vi "Weighted_Cross_Moments_TF.vi"(0 "Cluster 1":T1={"Colour"=0, "Inst type"=enum."Pitot-static tube", "Inst name"="Manometer voltage", "Symbol"="U", "Code name"="", "Extra Info"="U", "Inst Array"=enum."PWA", "Index"=0, "Voltage Index"=0, "Extra Titles"=[], "Extra Values"=[], "Eng Values"=[], "Time (ms)"=[], "TT / Voltage"=[], "U"=0.0, "u^2"=0.0, "u^3"=0.0, "u^4"=0.0, "Skew_u"=0.0, "Kurt_u"=0.0, "Mean % Err"=0.0, "% u'/U"=0.0} {"Skew_u" format="%.2f"; "% u'/U" format="%.2f"; "Mean % Err" format="%.2f"; "Kurt_u" format="%.2f"; "u^4" format="%.2f"; "u^3" format="%.2f"; "U" format="%.2f"; "u^2" format="%.2f"}, 1 "Cluster 2":T1={"Colour"=0, "Inst type"=enum."Pitot-static tube", "Inst name"="Manometer voltage", "Symbol"="U", "Code name"="", "Extra Info"="U", "Inst Array"=enum."PWA", "Index"=0, "Voltage Index"=0, "Extra Titles"=[], "Extra Values"=[], "Eng Values"=[], "Time (ms)"=[], "TT / Voltage"=[], "U"=0.0, "u^2"=0.0, "u^3"=0.0, "u^4"=0.0, "Skew_u"=0.0, "Kurt_u"=0.0, "Mean % Err"=0.0, "% u'/U"=0.0} {"Skew_u" format="%.2f"; "% u'/U" format="%.2f"; "Mean % Err" format="%.2f"; "Kurt_u" format="%.2f"; "u^4" format="%.2f"; "u^3" format="%.2f"; "U" format="%.2f"; "u^2" format="%.2f"}, 5 "Shift in":dbl[](array[numeric]) format="%.2f") -> (14 "Headers":string[](array[string]), 15 "Results":string[](array[string]), 19 "Shift out":dbl[](array[numeric]) format="%.2f")   [LabVIEW 2011]
uses:
  Controls/Analysis_info_cluster.ctl
  Controls/Inst_type.ctl
  Controls/Instrument_Array.ctl
  Globals/Meas_global.vi
panel:
  out "appended array":string[][](array[string])
  in  "Publish all results?":bool=TRUE
  in  "interp. method":i32(ring) items=["nearest", "linear", "spline", "cubic Hermite", "Lagrange"]
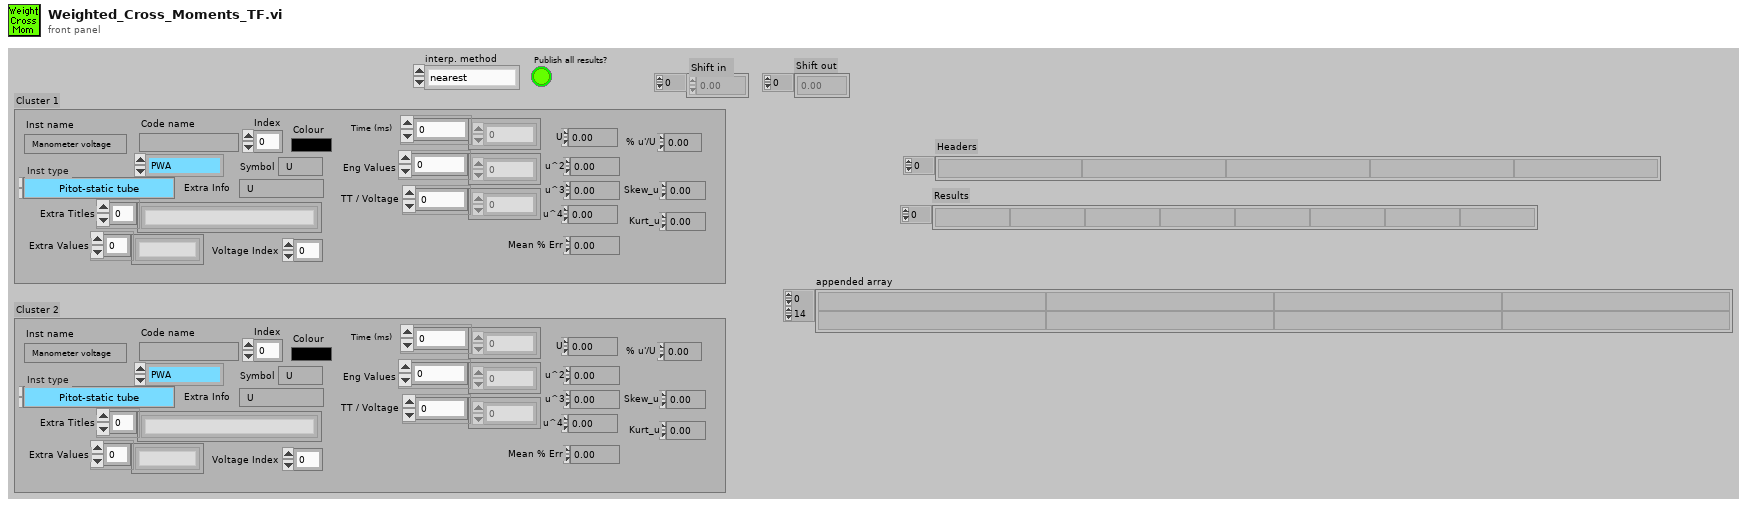
[diagram p1: front panel]
types:
  T1 = typedef "Analysis_info_cluster.ctl" = cluster{"Colour":u32, "Inst type":T2, "Inst name":string, "Symbol":string, "Code name":string, "Extra Info":string, "Inst Array":T3, "Index":i32, "Voltage Index":i32, "Extra Titles":string[], "Extra Values":string[], "Eng Values":dbl[], "Time (ms)":dbl[], "TT / Voltage":dbl[], "U":dbl, "u^2":dbl, "u^3":dbl, "u^4":dbl, "Skew_u":dbl, "Kurt_u":dbl, "Mean % Err":dbl, "% u'/U":dbl}
  T2 = typedef "Inst_type.ctl" = enum16{"Propeller anemometer", "Raw voltage", "Pressure Transducer", "Pitot-static tube", "Preston tube", "Hot wire", "Cross wire 1", "Cross wire 2", "Generic Linear", "Generic Polynomial", "Generic BackPoly", "Fast FID", "Thermocouple", "Cold wire", "Pulsed Wire", "LDA Vel", "LDA Tran time", "LDA Arr time"}
  T3 = typedef "Instrument_Array.ctl" = enum16{"PWA", "LDA", "Analogue"}
  T4 = enum16{"Mean only", "2nd Order Stats", "4th Order Stats"}
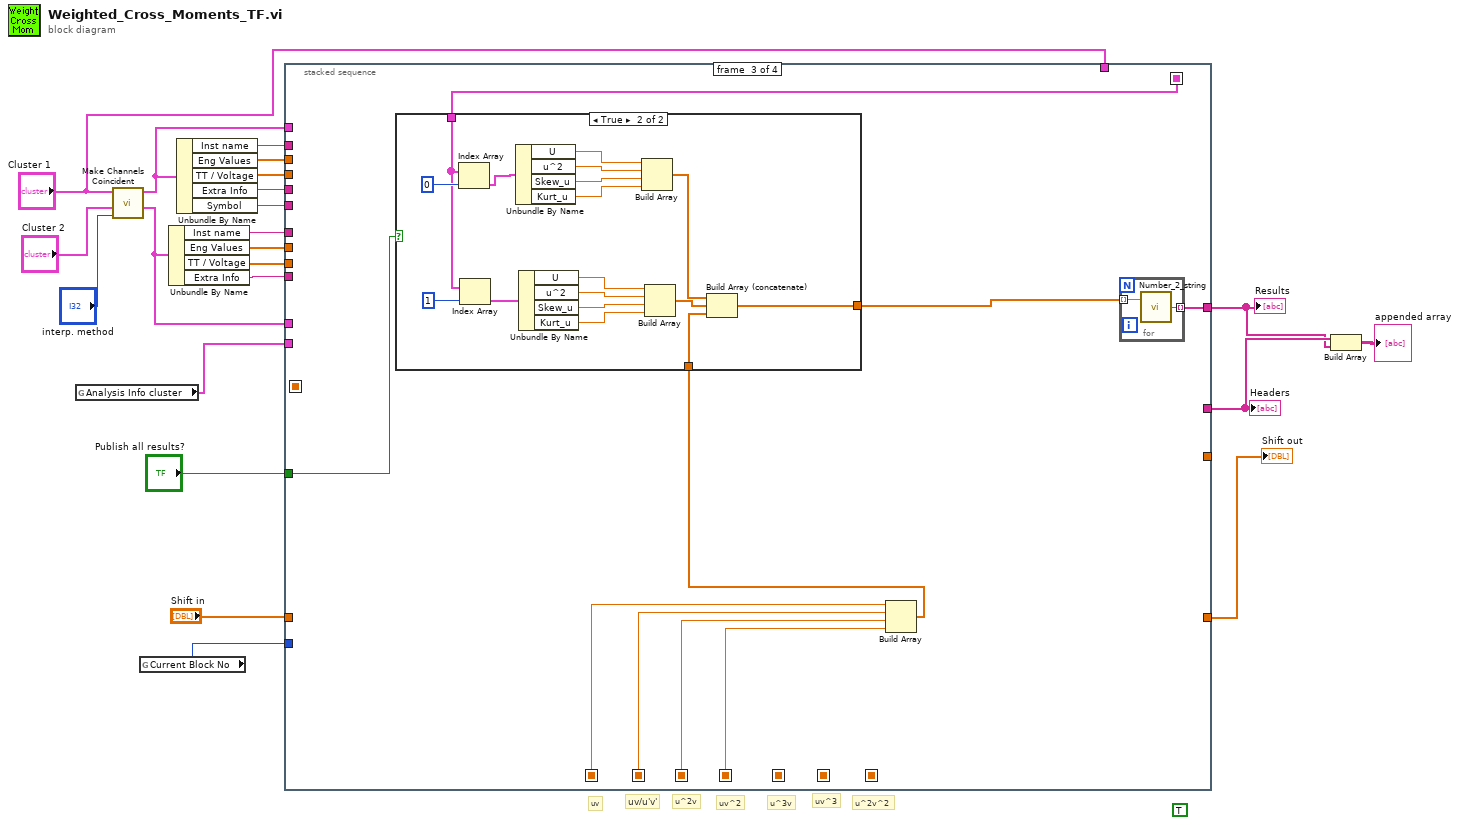
[diagram p0: block diagram]
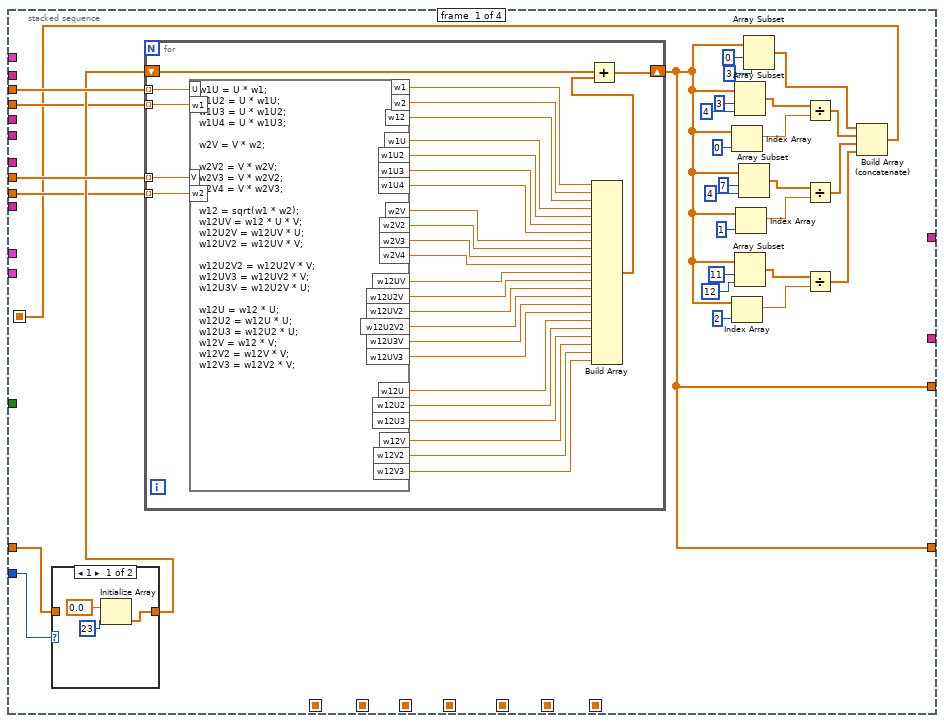
[diagram p2: hidden frame]
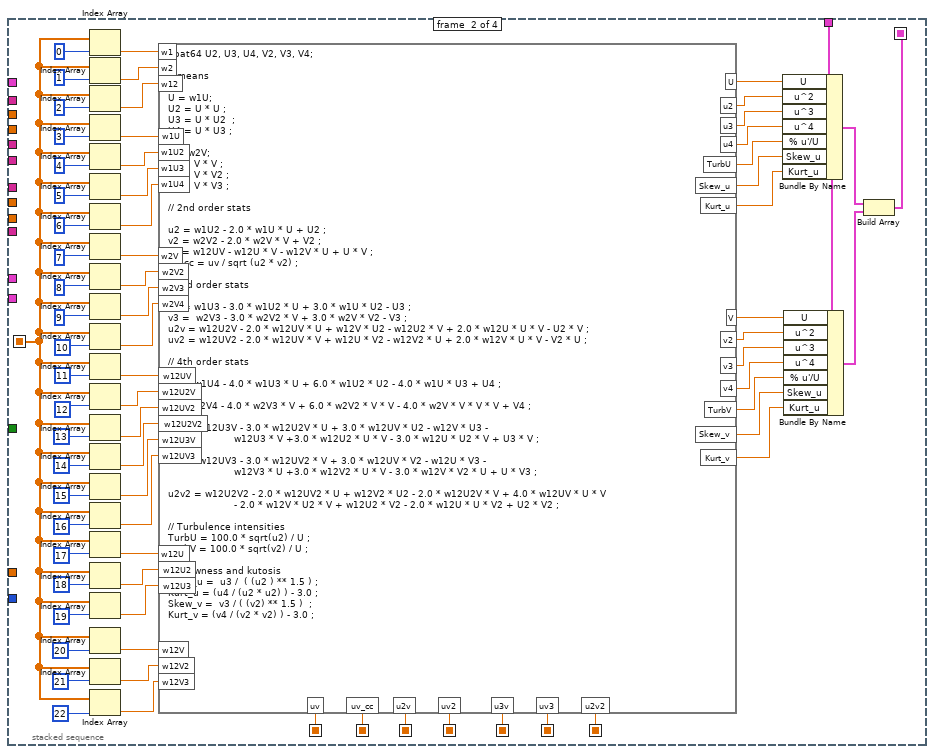
[diagram p4: hidden frame]
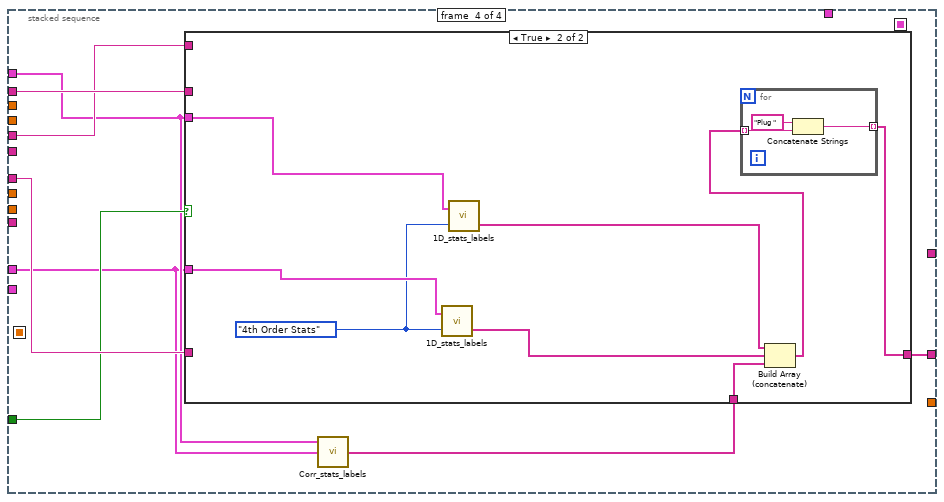
[diagram p6: hidden frame]
diagram:
  (unwired) TRUE
  # "u^2v^2"
  # "uv^3"
  # "u^3v"
  # "uv^2"
  # "u^2v"
  # "uv/u'v'"
  # "uv"
  n1 = global read "Meas_global.vi" "Analysis Info cluster"() -> (w18:T1[])
  n2 = call "Make Channels Coincident.vi"("interp. method"="interp. method", "Cluster 2"="Cluster 2", "Cluster 1"="Cluster 1") -> ("Coincident Channel 2"=w1:T1, "Coincident Channel 1"=w2:T1)  [unwired: 7 in]
  n3 = global read "Meas_global.vi" "Current Block No"() -> (w6:i32)
  n4 = Unbundle By Name(w1) -> ("Inst name"=w14:string, "Eng Values"=w20:dbl[], "TT / Voltage"=w21:dbl[], "Extra Info"=w17:string)
  n5 = Unbundle By Name(w2) -> ("Inst name"=w15:string, "Eng Values"=w19:dbl[], "TT / Voltage"=w22:dbl[], "Extra Info"=w16:string, "Symbol"=w3:string)
  n6 = stacked-sequence {
    seq-local: [_ w146 _ _] -> [_ _ w167 _]
    seq-local: [_ w145 _ _] -> [_ _ w166 _]
    seq-local: [w45 _ _ _] -> [_ w91 _ _]
    seq-local: [_ w140 _ _] -> [_ _ w165 _]
    seq-local: [_ w139 _ _] -> [_ _ w164 _]
    seq-local: [_ w87 _ _] -> [_ _ w162 _]
    seq-local: [_ w104 _ _] -> [_ _ _ _]
    seq-local: [_ w103 _ _] -> [_ _ _ _]
    seq-local: [_ w102 _ _] -> [_ _ _ _]
    tunnel: w19 -> [w52 _ _ _]
    tunnel: [w44 _ _ _] -> _
    tunnel: "Shift in" -> [w49 _ _ _]
    tunnel: w20 -> [w51 _ _ _]
    tunnel: w18 -> [_ _ _ _]
    tunnel: [_ _ w163 _] -> w7
    tunnel: w6 -> [w50 _ _ _]
    tunnel: w22 -> [w47 _ _ _]
    tunnel: w21 -> [w46 _ _ _]
    tunnel: "Cluster 1" -> [_ w107 _ _]
    tunnel: w17 -> [_ _ _ _]
    tunnel: w16 -> [_ _ _ w192]
    tunnel: [_ _ _ w194] -> w8
    tunnel: w15 -> [_ _ _ w193]
    tunnel: w14 -> [_ _ _ w195]
    tunnel: "Publish all results?" -> [_ _ w159 w191]
    tunnel: [w44 _ _ _] -> w5
    tunnel: w3 -> [_ _ _ _]
    tunnel: w2 -> [_ _ _ w190]
    tunnel: w1 -> [_ _ _ w189]
    frame #0 {
      n7 = case shown="1" w50 {
        tunnel: [w53 w56] -> w48
        tunnel: w49 -> [_ w56]
        frame 1 {
          n8 = Initialize Array(0.0 ("Element Data"), 23 ("Dimension Size")) -> (w53:dbl[])
        }
        frame 2, Default {
        }
      }
      n9 = for {
        shift-right: [w82] -> w44
        shift-left: w48 -> [w86]
        tunnel: w47 -> [w81] mode=indexing
        tunnel: w52 -> [w84] mode=indexing
        tunnel: w51 -> [w83] mode=indexing
        tunnel: w46 -> [w80] mode=indexing
        n10 = formula code="w1U = U * w1;\nw1U2 = U * w1U;\nw1U3 = U * w1U2;\nw1U4 = U * w1U3;\n\nw2V = V * w2;\n\nw2V2 = V * w2V;\nw2V3 = V * w2V2;\nw2V4 = V * w2V3;\n\nw12 = sqrt(w1 * w2);\nw12UV = w12 * U * V;\nw12U2V = w12UV * U;\nw12UV2 = w12UV * V;\n\nw12U2V2 = w12U2V * V;\nw12UV3 = w12UV2 * V;\nw12U3V = w12U2V * U;\n\nw12U = w12 * U;\nw12U2 = w12U * U;\nw12U3 = w12U2 * U;\nw12V = w12 * V;\nw12V2 = w12V * V;\nw12V3 = w12V2 * V;"("V"=w83, "U"=w84, "w1"=w81, "w2"=w80) -> ("w12UV"=w71:dbl, "w1U"=w79:dbl, "w2V"=w75:dbl, "w1U2"=w78:dbl, "w2V2"=w74:dbl, "w12U2V"=w70:dbl, "w12UV2"=w69:dbl, "w1U3"=w77:dbl, "w1U4"=w76:dbl, "w2V3"=w73:dbl, "w2V4"=w72:dbl, "w12U3V"=w67:dbl, "w12UV3"=w66:dbl, "w12U2V2"=w68:dbl, "w12U"=w62:dbl, "w12U2"=w61:dbl, "w12U3"=w60:dbl, "w12V"=w59:dbl, "w12V2"=w58:dbl, "w12V3"=w57:dbl, "w12"=w65:dbl, "w1"=w64:dbl, "w2"=w63:dbl)
        n11 = Build Array(w64, w63, w65, w79, w78, w77, w76, w75, w74, w73, w72, w71, w70, w69, w68, w67, w66, w62, w61, w60, w59, w58, w57) -> (w85:dbl[])
        n12 = Add(x=w86, y=w85) -> (x+y=w82:dbl[])
      }
      n13 = Index Array(array=w44, index=0 ("Index")) -> (element=w40:dbl)
      n14 = Index Array(array=w44, index=2 ("Index")) -> (element=w30:dbl)
      n15 = Array Subset(array=w44, index=3 ("Array Index"), length=4) -> (w41:dbl[])
      n16 = Array Subset(array=w44, index=11 ("Array Index"), length=12) -> (w31:dbl[])
      n17 = Index Array(array=w44, index=1 ("Index")) -> (element=w37:dbl)
      n18 = Array Subset(array=w44, index=7 ("Array Index"), length=4) -> (w36:dbl[])
      n19 = Array Subset(array=w44, index=0, length=3) -> (w23:dbl[])
      n20 = Divide(x=w41, y=w40) -> (x/y=w28:dbl[])
      n21 = Divide(x=w36, y=w37) -> (x/y=w27:dbl[])
      n22 = Divide(x=w31, y=w30) -> (x/y=w26:dbl[])
      n23 = Build Array (concatenate)(w23, w28, w27, w26) -> (w45:dbl[])
    }
    frame #1 {
      n24 = Index Array(array=w91, index=0) -> (element=w152:dbl)
      n25 = Index Array(array=w91, index=1) -> (element=w151:dbl)
      n26 = Index Array(array=w91, index=2) -> (element=w150:dbl)
      n27 = Index Array(array=w91, index=3) -> (element=w149:dbl)
      n28 = Index Array(array=w91, index=4) -> (element=w148:dbl)
      n29 = Index Array(array=w91, index=5) -> (element=w147:dbl)
      n30 = Index Array(array=w91, index=6) -> (element=w142:dbl)
      n31 = Index Array(array=w91, index=7) -> (element=w141:dbl)
      n32 = Index Array(array=w91, index=8) -> (element=w132:dbl)
      n33 = Index Array(array=w91, index=9) -> (element=w131:dbl)
      n34 = Index Array(array=w91, index=10) -> (element=w134:dbl)
      n35 = Index Array(array=w91, index=11) -> (element=w133:dbl)
      n36 = Index Array(array=w91, index=12) -> (element=w115:dbl)
      n37 = Index Array(array=w91, index=13) -> (element=w114:dbl)
      n38 = Index Array(array=w91, index=14) -> (element=w110:dbl)
      n39 = Index Array(array=w91, index=15) -> (element=w109:dbl)
      n40 = Index Array(array=w91, index=16) -> (element=w108:dbl)
      n41 = Index Array(array=w91, index=17) -> (element=w97:dbl)
      n42 = Index Array(array=w91, index=18) -> (element=w96:dbl)
      n43 = Index Array(array=w91, index=19) -> (element=w95:dbl)
      n44 = Index Array(array=w91, index=20) -> (element=w94:dbl)
      n45 = Index Array(array=w91, index=21) -> (element=w90:dbl)
      n46 = Index Array(array=w91, index=22) -> (element=w89:dbl)
      n47 = formula code="float64 U2, U3, U4, V2, V3, V4;\n\n// means\n\nU = w1U;\nU2 = U * U ;\nU3 = U * U2  ;\nU4 = U * U3 ;\n\nV = w2V;\nV2 = V * V ;\nV3 = V * V2 ;\nV4 = V * V3 ;\n\n// 2nd order stats\n\nu2 = w1U2 - 2.0 * w1U * U + U2 ;\nv2 = w2V2 - 2.0 * w2V * V + V2 ;\nuv = w12UV - w12U * V - w12V * U + U * V ;\nuv_cc = uv / sqrt (u2 * v2) ;\n\n// 3rd order stats\n\nu3 = w1U3 - 3.0 * w1U2 * U + 3.0 * w1U * U2 - U3 ;\nv3 =  w2V3 - 3.0 * w2V2 * V + 3.0 * w2V * V2 - V3 ;\nu2v = w12U2V - 2.0 * w12UV * U + w12V * U2 - w12U2 * V + 2.0 * w12U * U * V - U2 * V ;\nuv2 = w12UV2 - 2.0 * w12UV * V + w12U * V2 - w12V2 * U + 2.0 * w12V * U * V - V2 * U ;\n\n// 4th order stats\n\nu4 = w1U4 - 4.0 * w1U3 * U + 6.0 * w1U2 * U2 - 4.0 * w1U * U3 + U4 ;\n\nv4 = w2V4 - 4.0 * w2V3 * V + 6.0 * w2V2 * V * V - 4.0 * w2V * V * V * V + V4 ;\n\nu3v = w12U3V - 3.0 * w12U2V * U + 3.0 * w12UV * U2 - w12V * U3 - \n                      w12U3 * V +3.0 * w12U2 * U * V - 3.0 * w12U * U2 * V + U3 * V ;\n\nuv3 = w12UV3 - 3.0 * w12UV2 * V + 3.0 * w12UV * V2 - w12U * V3 - \n                      w12V3 * U +3.0 * w12V2 * U * V - 3.0 * w12V * V2 * U + U * V3 ;\n\nu2v2 = w12U2V2 - 2.0 * w12UV2 * U + w12V2 * U2 - 2.0 * w12U2V * V + 4.0 * w12UV * U * V\n                      - 2.0 * w12V * U2 * V + w12U2 * V2 - 2.0 * w12U * U * V2 + U2 * V2 ; \n\n// Turbulence intensities\nTurbU = 100.0 * sqrt(u2) / U ;\nTurbV = 100.0 * sqrt(v2) / U ;\n\n// Skewness and kutosis\nSkew_u =  u3 /  ( (u2 ) ** 1.5 ) ;\nKurt_u = (u4 / (u2 * u2) ) - 3.0 ;\nSkew_v =  v3 / ( (v2) ** 1.5 )  ;\nKurt_v = (v4 / (v2 * v2) ) - 3.0 ;"("w1"=w152, "w2"=w151, "w12"=w150, "w1U2"=w148, "w1U3"=w147, "w1U"=w149, "w1U4"=w142, "w2V"=w141, "w2V2"=w132, "w2V4"=w134, "w2V3"=w131, "w12UV"=w133, "w12U2V"=w115, "w12UV2"=w114, "w12U2V2"=w110, "w12U3V"=w109, "w12UV3"=w108, "w12U2"=w96, "w12U3"=w95, "w12V"=w94, "w12V2"=w90, "w12U"=w97, "w12V3"=w89) -> ("uv"=w146:dbl, "U"=w124:dbl, "V"=w129:dbl, "u2"=w121:dbl, "v2"=w128:dbl, "uv_cc"=w145:dbl, "u2v"=w140:dbl, "uv2"=w139:dbl, "u3"=w122:dbl, "u4"=w123:dbl, "v3"=w127:dbl, "v4"=w126:dbl, "TurbU"=w130:dbl, "TurbV"=w125:dbl, "Skew_v"=w118:dbl, "Skew_u"=w119:dbl, "Kurt_u"=w106:dbl, "Kurt_v"=w105:dbl, "u3v"=w104:dbl, "uv3"=w103:dbl, "u2v2"=w102:dbl)
      n48 = Bundle By Name(cluster=w107, "U"=w124, "u^2"=w121, "u^3"=w122, "u^4"=w123, "% u'/U"=w130, "Skew_u"=w119, "Kurt_u"=w106) -> (w88:T1)
      n49 = Bundle By Name(cluster=w107, "U"=w129, "u^2"=w128, "u^3"=w127, "u^4"=w126, "% u'/U"=w125, "Skew_u"=w118, "Kurt_u"=w105) -> (w120:T1)
      n50 = Build Array(w88, w120) -> (w87:T1[])
    }
    frame #2 {
      n51 = Build Array(w167, w166, w165, w164) -> (w161:dbl[])
      n52 = case shown="True" w159 {
        tunnel: w162 -> [_ w184]
        tunnel: w161 -> [w168 w177]
        tunnel: [w168 w176] -> w160
        frame False {
        }
        frame True {
          n53 = Index Array(array=w184, index=0) -> (element=w170:T1)
          n54 = Index Array(array=w184, index=1) -> (element=w179:T1)
          n55 = Unbundle By Name(w170) -> ("U"=w174:dbl, "u^2"=w173:dbl, "Skew_u"=w172:dbl, "Kurt_u"=w171:dbl)
          n56 = Unbundle By Name(w179) -> ("U"=w175:dbl, "u^2"=w180:dbl, "Skew_u"=w181:dbl, "Kurt_u"=w182:dbl)
          n57 = Build Array(w174, w173, w172, w171) -> (w169:dbl[])
          n58 = Build Array(w175, w180, w181, w182) -> (w178:dbl[])
          n59 = Build Array (concatenate)(w169, w178, w177) -> (w176:dbl[])
        }
      }
      n60 = for {
        tunnel: w160 -> [w187] mode=indexing
        tunnel: [w186] -> w163 mode=indexing
        n61 = call "Number_2_string.vi"("number"=w187) -> ("String"=w186:string)  [unwired: 1 in]
      }
    }
    frame #3 {
      n62 = call "Corr_stats_labels.vi"("Inst 2 Units"=w189, "Inst 1 Units"=w190) -> ("Output"=w188:string[])  [unwired: 1 in]
      n63 = case shown="True" w191 {
        tunnel: w188 -> [w196 w204]
        tunnel: w195 -> [_ _]
        tunnel: [w196 w197] -> w194
        tunnel: w193 -> [_ _]
        tunnel: w192 -> [_ _]
        tunnel: w190 -> [_ w203]
        tunnel: w189 -> [_ w202]
        frame False {
        }
        frame True {
          w200 = T4."4th Order Stats" ("Mode selector")
          n64 = call "1D_stats_labels.vi"("Mode selector"=w200, "Analysis Info Cluster"=w202) -> ("Output"=w201:string[])  [unwired: 1 in]
          n65 = call "1D_stats_labels.vi"("Mode selector"=w200, "Analysis Info Cluster"=w203) -> ("Output"=w199:string[])  [unwired: 1 in]
          n66 = Build Array (concatenate)(w199, w201, w204) -> (w198:string[])
          n67 = for {
            tunnel: w198 -> [w207] mode=indexing
            tunnel: [w205] -> w197 mode=indexing
            n68 = Concatenate Strings("Plug " ("string"), w207) -> (w205:string)
          }
        }
      }
    }
  }
  "Shift out" <- w5
  "Headers" <- w8
  "Results" <- w7
  n69 = Build Array(w8, w7) -> (→"appended array":string[][])
